vi "批量读D+5个+32位.vi"(8 "error out":errorcluster, 10 "读取D地址":i32, 11 "VISA resource name out":refnum<visa-resource-name>) -> (0 "error IO":errorcluster, 1 "通讯延时":u32, 2 "数组":i32[](array[numeric]), 3 "VISA resource name out 2":refnum<visa-resource-name>)   [LabVIEW 2018]
uses:
  <vilib>/Instr/_visa.llb/VISA Configure Serial Port (Instr).vi
panel:
  out "连接的字符串 2":string
  out "连接的字符串":string
  out "读取缓冲区":string
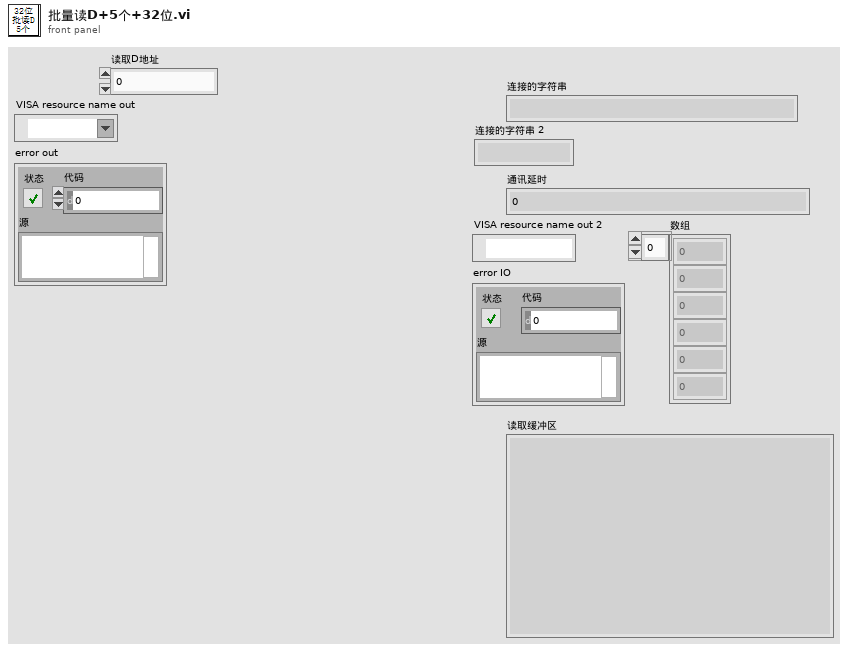
[diagram p1: front panel]
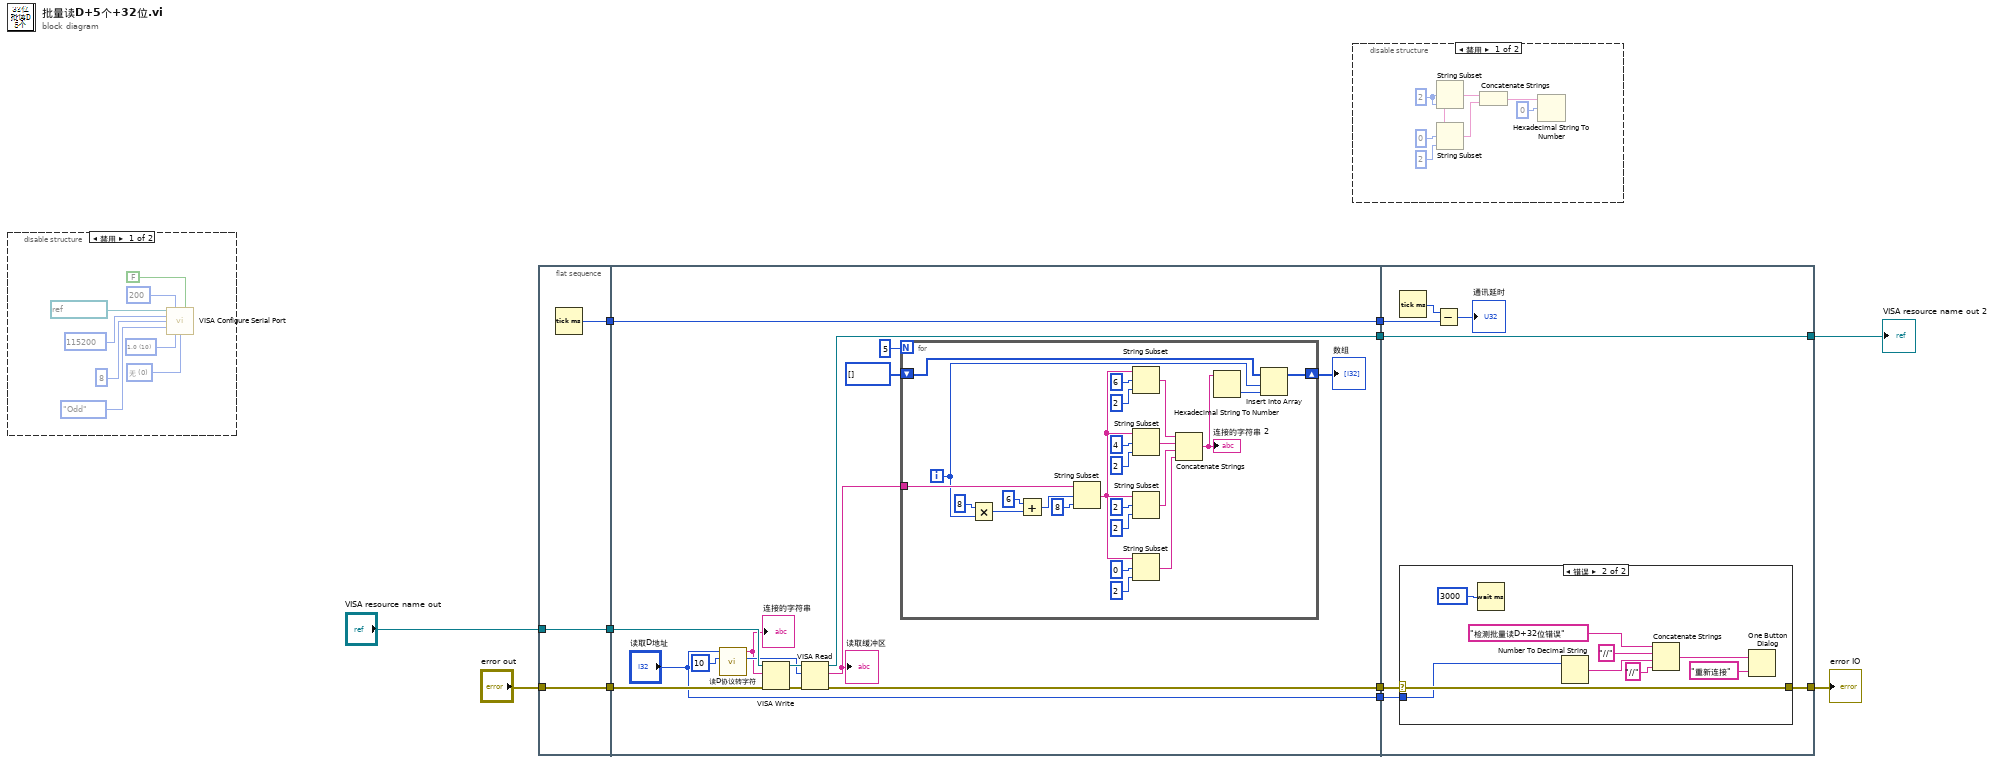
[diagram p0: block diagram]
diagram:
  n1 = disable-structure shown="禁用" {
    frame Disabled {
      w13 = u16 0 items=["无", "XON/XOFF", "RTS/CTS", "XON/XOFF & RTS/CTS", "DTR/DSR", "XON/XOFF & DTR/DSR"] ("flow control (0:none)")
      w14 = u16 10 items=["1.0"=10, "1.5"=15, "2.0"=20] ("stop bits (10: 1 bit)")
      n2 = call-poly "VISA Configure Serial Port"("VISA resource name"=refnum<visa-resource-name> "COM3", "timeout (10sec)"=u32 200, "Enable Termination\nChar (T)"=FALSE ("Enable Termination\nChar (T)"), "baud rate (9600)"=u32 115200, "data bits (8)"=u16 8, "parity (0:none)"=enum16{"None", "Odd", "Even", "Mark", "Space"}."Odd", "stop bits (10: 1 bit)"=w14, "flow control (0:none)"=w13) -> ()  [unwired: 6 in, 2 out]
    }
    frame Enabled {
    }
  }
  n3 = flat-sequence {
    tunnel: [w22] -> w11
    tunnel: "VISA resource name out" -> [w21]
    tunnel: [w21] -> w10
    tunnel: [w20] -> w9
    tunnel: "error out" -> [w20]
    tunnel: w11 -> [w37]
    tunnel: [w37] -> w8
    tunnel: [w36] -> w7
    tunnel: [w35] -> w6
    tunnel: w10 -> [w34]
    tunnel: w9 -> [w33]
    tunnel: ["读取D地址"] -> w1
    tunnel: w8 -> [w67]
    tunnel: w7 -> [w65]
    tunnel: [w65] -> w3
    tunnel: w6 -> [w64]
    tunnel: [w63] -> w2
    tunnel: w1 -> [w62]
    frame #0 {
      n4 = Tick Count (ms)() -> (millisecond timer value=w22:u32)
    }
    frame #1 {
      n5 = call "读D协议转字符.vi"("读取D个数"=10, "读取D地址"="读取D地址") -> ("读取的字节数"=w30:i32, "连接的字符串"=w29:string)  [unwired: 8 in]
      "连接的字符串" <- w29
      n6 = VISA Write(VISA resource name=w34, write buffer=w29, error in (no error)=w33) -> (VISA resource name out=w32:refnum<visa-resource-name>, error out=w31:errorcluster)  [unwired: 1 out]
      n7 = VISA Read(VISA resource name=w32, byte count=w30, error in (no error)=w31) -> (VISA resource name out=w36:refnum<visa-resource-name>, read buffer=w28:string, error out=w35:errorcluster)  [unwired: 1 out]
      "读取缓冲区" <- w28
      n8 = for {
        N: 5 -> [_]
        tunnel: w28 -> [w61]
        shift-right: [w57] -> w24
        shift-left: i32[] [] -> [w58]
        i -> [w42]
        n9 = Multiply(x=8, y=w42) -> (x*y=w39:i32)
        n10 = Add(x=6 ("偏移量(0)"), y=w39) -> (x+y=w38:i32)
        n11 = String Subset(string=w61, offset (0)=w38, length (rest)=8 ("长度（剩余）")) -> (substring=w60:string)
        n12 = String Subset(string=w60, offset (0)=6 ("偏移量(0)"), length (rest)=2 ("长度（剩余）")) -> (substring=w52:string)
        n13 = String Subset(string=w60, offset (0)=4 ("偏移量(0)"), length (rest)=2 ("长度（剩余）")) -> (substring=w51:string)
        n14 = String Subset(string=w60, offset (0)=2 ("偏移量(0)"), length (rest)=2 ("长度（剩余）")) -> (substring=w50:string)
        n15 = String Subset(string=w60, offset (0)=0 ("偏移量(0)"), length (rest)=2 ("长度（剩余）")) -> (substring=w49:string)
        n16 = Concatenate Strings(w52, w51, w50, w49) -> (w48:string)
        "连接的字符串 2" <- w48
        n17 = Hexadecimal String To Number(string=w48) -> (number=w59:u32)  [unwired: 2 in, 1 out]
        n18 = Insert Into Array(array=w58, index=w42, new element=w59) -> (w57:i32[])
      }
      "数组" <- w24
    }
    frame #2 {
      n19 = Tick Count (ms)() -> (millisecond timer value=w68:u32)
      n20 = case shown="错误" w64 {
        selector: w64 -> [w69 w78]
        tunnel: [w69 w78] -> w63
        tunnel: w62 -> [_ w72]
        frame No Error {
        }
        frame Error {
          n21 = Wait (ms)(milliseconds to wait=u32 3000 ("等待时间（毫秒）")) -> ()  [unwired: 1 out]
          n22 = Number To Decimal String(number=w72) -> (decimal integer string=w71:string)  [unwired: 1 in]
          n23 = Concatenate Strings("检测批量读D+32位错误" ("消息"), "//" ("字符串"), w71, "//" ("字符串")) -> (w70:string)
          n24 = One Button Dialog(message=w70, button name ("OK")="重新连接" ("按钮名称（“确定”）")) -> ()  [unwired: 1 out]
        }
      }
      n25 = Subtract(x=w68, y=w67) -> (x-y=→"通讯延时":u32)
    }
  }
  n26 = disable-structure shown="禁用" {
    frame Disabled {
      w82 = 2 ("偏移量(0)")
      n27 = String Subset(offset (0)=0 ("偏移量(0)"), length (rest)=2 ("长度（剩余）")) -> (string=w81:string, substring=w83:string)
      n28 = String Subset(string=w81, offset (0)=w82, length (rest)=w82) -> (substring=w84:string)
      n29 = Concatenate Strings(w84, w83) -> (w85:string)
      n30 = Hexadecimal String To Number(string=w85, offset=0 ("偏移量")) -> ()  [unwired: 1 in, 2 out]
    }
    frame Enabled {
    }
  }
  "VISA resource name out 2" <- w3
  "error IO" <- w2
